vi "ContextHelp_StartPopUpTask.vi"(1 "CallerRef":refnum<vi>, 5 "error in (no error)":errorcluster) -> (14 "PopUpTaskEvent":T1, 19 "error out":errorcluster)   [LabVIEW 2020]
uses:
  <resource>/Framework/Providers/Open_GDS/UML/ContextHelp/ContextHelp_EventType.ctl
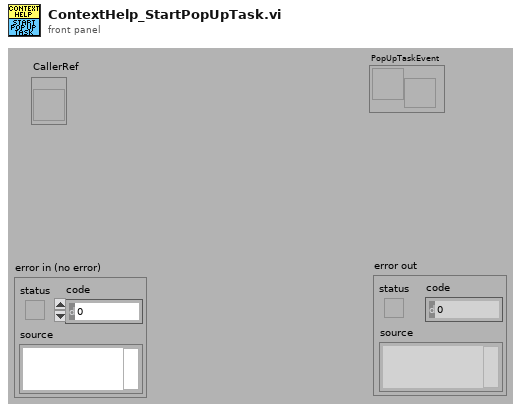
[diagram p1: front panel]
types:
  T1 = typedef "ContextHelp_EventType.ctl" = refnum<user-event>
  T2 = enum16{"SetPopUpEventTask", "GetStatus", "SetOpenState"}
  T3 = enum32{"Bad", "Idle", "Run top level", "Running"}
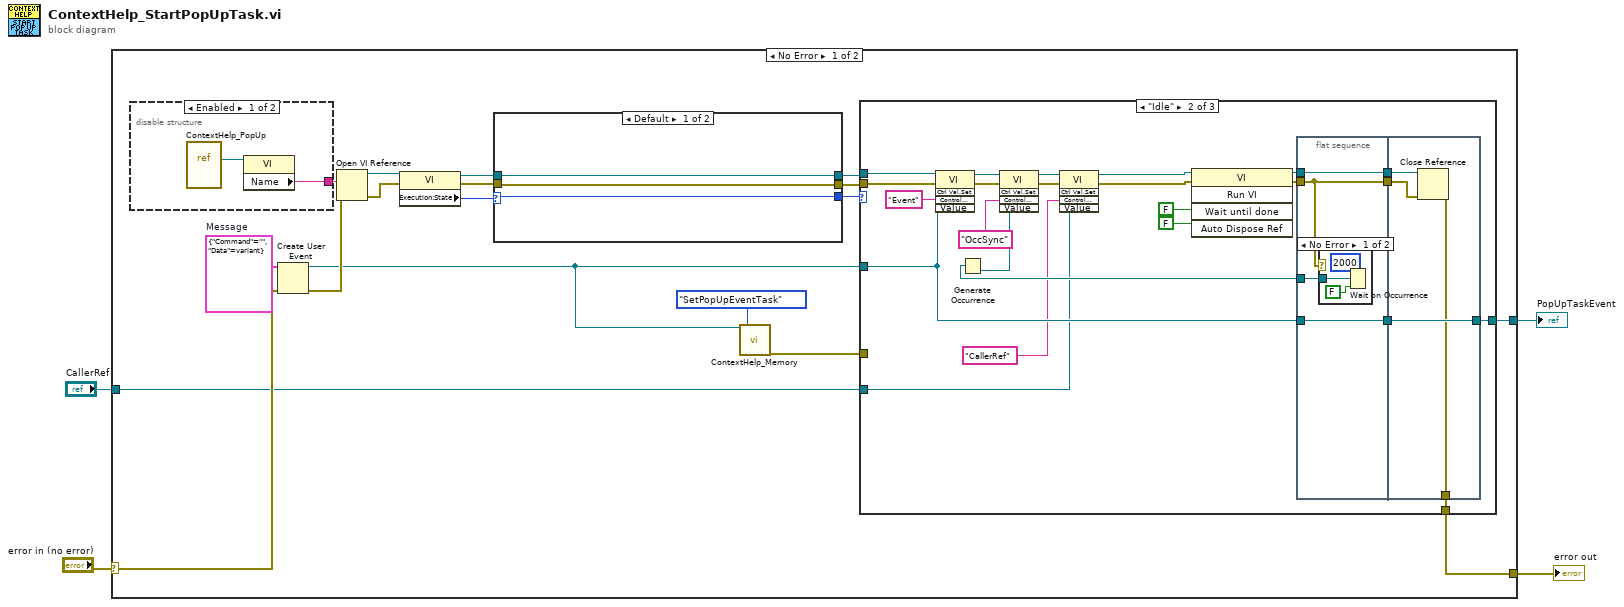
[diagram p0: block diagram]
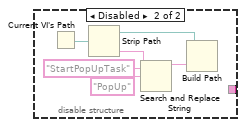
[diagram p2: hidden frame]
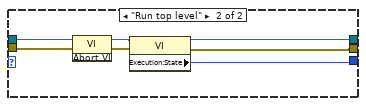
[diagram p3: hidden frame]
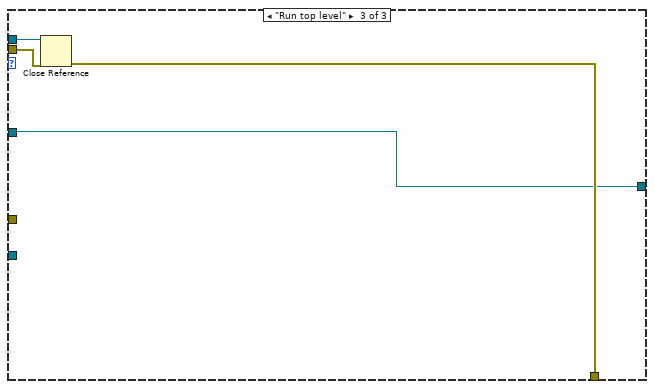
[diagram p6: hidden frame]
diagram:
  n1 = case shown="No Error" "error in (no error)" {
    selector: "error in (no error)" -> [w18 w81]
    tunnel: [w21 _] -> w4
    tunnel: [w20 w81] -> w3
    tunnel: "CallerRef" -> [w9 _]
    frame No Error {
      w22 = cluster{"Command":string, "Data":variant} {"Command"="", "Data"=variant}  # Message
      n2 = disable-structure shown="Enabled" {
        disable-tunnel: [w23 _] -> w5
        frame Enabled {
          n3 = vi-ref <resource>:"ContextHelp_PopUp.vi"() -> (w24:refnum<vi>)
          n4 = property class="VI"(reference=w24) -> ("Name"=w23:string)  [unwired: 1 in, 2 out]
        }
        frame Disabled {
          n5 = Current VI's Path() -> (path=w30:path)
          n6 = Strip Path(path=w30) -> (stripped path=w27:path, name=w29:string)
          n7 = Search and Replace String(input string=w29, search string="StartPopUpTask", replace string="PopUp" ("replace string (\"\")")) -> (result string=w28:string)  [unwired: 1 in, 7 out]
          n8 = Build Path(base path=w27, name or relative path=w28) -> ()  [unwired: 1 out]
        }
      }
      n9 = Create User Event(user event datatype=w22, error in=w18) -> (user event=w7:refnum<user-event>, error out=w19:errorcluster)
      n10 = Open VI Reference(vi path=w5, error in (no error)=w19) -> (vi reference=w17:refnum<vi>, error out=w16:errorcluster)  [unwired: 4 out]
      n11 = property class="VI"(reference=w17, error in=w16) -> (reference out=w15:refnum<vi>, error out=w14:errorcluster, "Execution:State"=w13:T3)
      n12 = case shown="Default" w13 {
        selector: w13 -> [w33 _]
        tunnel: w15 -> [w31 w40]
        tunnel: w14 -> [w32 w39]
        tunnel: [w33 w36] -> w12
        tunnel: [w32 w34] -> w11
        tunnel: [w31 w35] -> w10
        frame Default {
        }
        frame "Run top level" {
          n13 = invoke class="VI" method="Abort VI"(reference=w40, error in=w39) -> (reference out=w38:refnum<vi>, error out=w37:errorcluster)  [unwired: 1 in, 1 out]
          n14 = property class="VI"(reference=w38, error in=w37) -> (reference out=w35:refnum<vi>, error out=w34:errorcluster, "Execution:State"=w36:T3)
        }
      }
      n15 = call <resource>:"ContextHelp_Memory.vi"("PopUpTaskEvent"=w7, "Actio(GetStatus)n"=T2."SetPopUpEventTask") -> ("error out"=w6:errorcluster)  [unwired: 2 in, 15 out]
      n16 = case shown="\"Idle\"" w12 {
        tunnel: w10 -> [_ w62 w80]
        tunnel: w11 -> [w41 w61 w79]
        tunnel: w7 -> [w42 w51 w77]
        tunnel: [w42 w50 w77] -> w21
        tunnel: [w41 w49 w78] -> w20
        tunnel: w9 -> [_ w45 _]
        tunnel: w6 -> [_ _ _]
        frame "Bad", Default {
        }
        frame "Idle" {
          n17 = invoke class="VI" method="Ctrl Val.Set"(reference=w62, error in=w61, "Control Name"="Event", "Value"=w51) -> (reference out=w55:refnum<vi>, error out=w54:errorcluster)  [unwired: 1 in, 3 out]
          n18 = Generate Occurrence() -> (w52:refnum<k4>)
          n19 = invoke class="VI" method="Ctrl Val.Set"(reference=w55, error in=w54, "Control Name"="OccSync", "Value"=w52) -> (reference out=w48:refnum<vi>, error out=w47:errorcluster)  [unwired: 1 in, 3 out]
          n20 = invoke class="VI" method="Ctrl Val.Set"(reference=w48, error in=w47, "Control Name"="CallerRef", "Value"=w45) -> (reference out=w43:refnum<vi>, error out=w44:errorcluster)  [unwired: 1 in, 3 out]
          n21 = invoke class="VI" method="Run VI"(reference=w43, error in=w44, "Wait until done"=FALSE, "Auto Dispose Ref"=FALSE) -> (reference out=w57:refnum<vi>, error out=w56:errorcluster)  [unwired: 1 in, 3 out]
          n22 = flat-sequence {
            tunnel: w51 -> [w68]
            tunnel: w56 -> [w66]
            tunnel: w57 -> [w69]
            tunnel: [w69] -> w65
            tunnel: [w66] -> w64
            tunnel: [w68] -> w63
            tunnel: w52 -> [w67]
            tunnel: w65 -> [w76]
            tunnel: w64 -> [w75]
            tunnel: w63 -> [w74]
            tunnel: [w74] -> w50
            tunnel: [w73] -> w49
            frame #0 {
              n23 = case shown="No Error" w66 {
                tunnel: w67 -> [w72 _]
                frame No Error {
                  n24 = Wait on Occurrence(1:FALSE ("ignore previous (T)"), 2:w72, 3:2000 ("ms timeout (-1)")) -> ()  [unwired: 1 out]
                }
                frame Error {
                }
              }
            }
            frame #1 {
              n25 = Close Reference(reference=w76, error in (no error)=w75) -> (error out=w73:errorcluster)
            }
          }
        }
        frame "Run top level" {
          n26 = Close Reference(reference=w80, error in (no error)=w79) -> (error out=w78:errorcluster)
        }
      }
    }
    frame Error {
    }
  }
  "PopUpTaskEvent" <- w4
  "error out" <- w3
